vi "Calculate_samples.vi"(4 "Olfactormeter parameters":T2) -> (1 "Samples":T1)   [LabVIEW 2016]
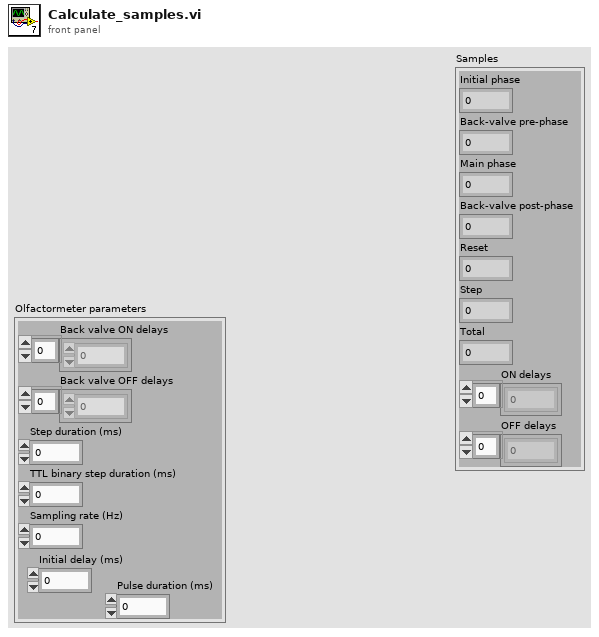
[diagram p1: front panel]
types:
  T1 = cluster{"Initial phase":i32, "Back-valve pre-phase ":i32, "Main phase":i32, "Back-valve post-phase":i32, "Reset":i32, "Step":i32, "Total":i32, "ON delays":i32[], "OFF delays":i32[]}
  T2 = cluster{"Back valve ON delays":dbl[], "Back valve OFF delays":dbl[], "Step duration (ms)":dbl, "TTL binary step duration (ms)":dbl, "Sampling rate (Hz)":dbl, "Initial delay (ms)":dbl, "Pulse duration (ms)":dbl}
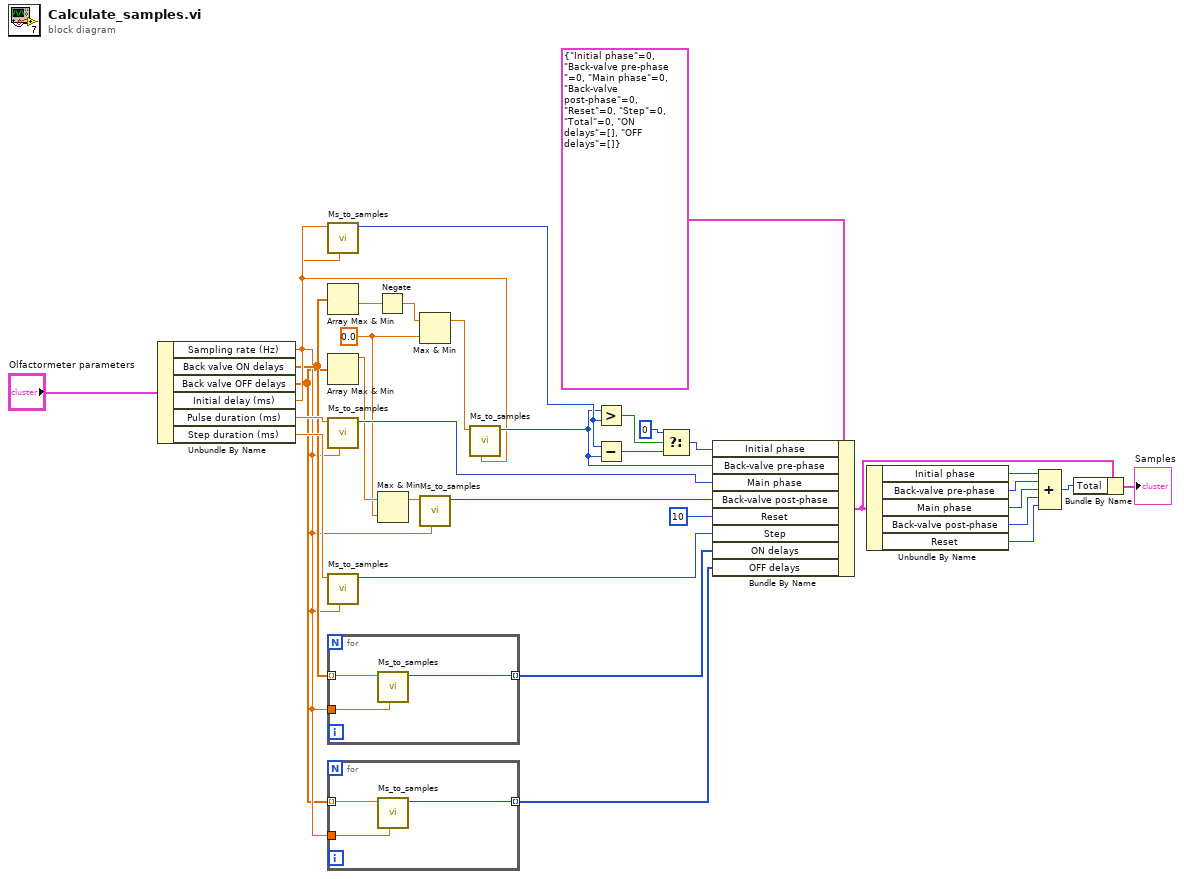
[diagram p0: block diagram]
diagram:
  w28 = 0.0 ("y")
  n1 = Unbundle By Name("Olfactormeter parameters") -> ("Sampling rate (Hz)"=w11:dbl, "Back valve ON delays"=w13:dbl[], "Back valve OFF delays"=w10:dbl[], "Initial delay (ms)"=w24:dbl, "Pulse duration (ms)"=w23:dbl, "Step duration (ms)"=w15:dbl)
  n2 = call "Ms_to_samples.vi"("Sampling rate (Hz)"=w11, "Step duration (ms)"=w24) -> ("Numeric"=w20:i32)  [unwired: 9 in]
  n3 = Array Max & Min(array=w13) -> (min value=w31:dbl)  [unwired: 3 out]
  n4 = Array Max & Min(array=w10) -> (max value=w29:dbl)  [unwired: 3 out]
  n5 = call "Ms_to_samples.vi"("Sampling rate (Hz)"=w11, "Step duration (ms)"=w23) -> ("Numeric"=w32:i32)  [unwired: 9 in]
  n6 = call "Ms_to_samples.vi"("Sampling rate (Hz)"=w11, "Step duration (ms)"=w15) -> ("Numeric"=w14:i32)  [unwired: 9 in]
  n7 = for {
    tunnel: w13 -> [w37] mode=indexing
    tunnel: w11 -> [w36]
    tunnel: [w35] -> w12 mode=indexing
    n8 = call "Ms_to_samples.vi"("Sampling rate (Hz)"=w36, "Step duration (ms)"=w37) -> ("Numeric"=w35:i32)  [unwired: 9 in]
  }
  n9 = for {
    tunnel: w10 -> [w40] mode=indexing
    tunnel: w11 -> [w39]
    tunnel: [w38] -> w9 mode=indexing
    n10 = call "Ms_to_samples.vi"("Sampling rate (Hz)"=w39, "Step duration (ms)"=w40) -> ("Numeric"=w38:i32)  [unwired: 9 in]
  }
  n11 = Negate(x=w31) -> (-x=w30:dbl)
  n12 = Max & Min(x=w29, y=w28) -> (max(x,y)=w27:dbl)  [unwired: 1 out]
  n13 = Max & Min(x=w30, y=w28) -> (max(x,y)=w22:dbl)  [unwired: 1 out]
  n14 = call "Ms_to_samples.vi"("Sampling rate (Hz)"=w11, "Step duration (ms)"=w27) -> ("Numeric"=w26:i32)  [unwired: 9 in]
  n15 = call "Ms_to_samples.vi"("Sampling rate (Hz)"=w11, "Step duration (ms)"=w22) -> ("Numeric"=w16:i32)  [unwired: 9 in]
  n16 = Greater?(x=w16, y=w20) -> (0:w21:bool)
  n17 = Subtract(x=w20, y=w16) -> (x-y=w19:i32)
  n18 = Select(t=0, s=w21, f=w19) -> (s? t:f=w18:i32)
  n19 = Bundle By Name(cluster=T1 {"Initial phase"=0, "Back-valve pre-phase "=0, "Main phase"=0, "Back-valve post-phase"=0, "Reset"=0, "Step"=0, "Total"=0, "ON delays"=[], "OFF delays"=[]}, "Initial phase"=w18, "Back-valve pre-phase"=w16, "Main phase"=w32, "Back-valve post-phase"=w26, "Reset"=10, "Step"=w14, "ON delays"=w12, "OFF delays"=w9) -> (w2:T1)
  n20 = Unbundle By Name(w2) -> ("Initial phase"=w8:i32, "Back-valve pre-phase"=w7:i32, "Main phase"=w6:i32, "Back-valve post-phase"=w5:i32, "Reset"=w4:i32)
  n21 = Compound Arithmetic op=ADD(w8, w7, w6, w5, w4) -> (w3:i32)
  n22 = Bundle By Name(cluster=w2, "Total"=w3) -> (→"Samples":T1)
